vi "Test_PreloadNormalMsg_SendLowPriorityStop_StopAfterNormalMsg.vi"(8 "error in (no error)":errorcluster, 11 "TestCase in":refnum<class "TestPriorityStopMessage.lvclass">) -> (0 "error out":errorcluster, 3 "TestCase out":refnum<class "TestPriorityStopMessage.lvclass">)   [LabVIEW 2017, in "TestPriorityStopMessage.lvclass"]
uses:
  TestPriorityStopMessage.lvclass
  <vilib>/ActorFramework/Message Enqueuer/Message Priority.ctl
  <vilib>/ActorFramework/Message Enqueuer/Message Enqueuer.lvclass/Message Enqueuer.ctl
  Doubles/MessageCountsExecutions/MessageCountsExecutions.lvclass
  C:/Program Files (x86)/National Instruments/LabVIEW 2017/vi.lib/ActorFramework/Message/Message.lvclass
  Doubles/ActorBlockedUntilNotified/ActorBlockedUntilNotified.lvclass
  C:/Program Files (x86)/National Instruments/LabVIEW 2017/vi.lib/ActorFramework/Actor/Actor.lvclass
  <vilib>/ActorFramework/Stop Msg/Stop Msg.lvclass
  <vilib>/ActorFramework/Message Priority Queue/Priority Enqueue.vi
  <vilib>/ActorFramework/Actor/Actor.lvclass
  <vilib>/ActorFramework/Message Enqueuer/Message Enqueuer.lvclass
  Source/PriorityStopMessage/PriorityStopMessage.lvclass
panel:
  out "Msg Notification History":cluster{u32, "timed out?":bool}[](array[cluster])
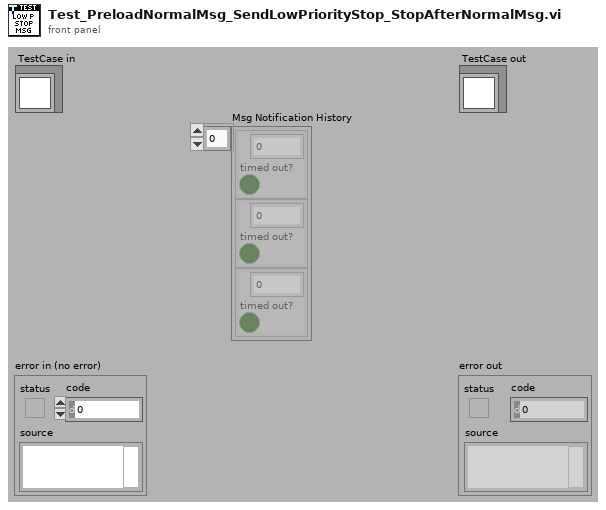
[diagram p1: front panel]
types:
  T1 = typedef "Actor Framework.lvlib/Message Enqueuer.lvclass/Message Priority.ctl" = enum16{"Low", "Normal", "High"}
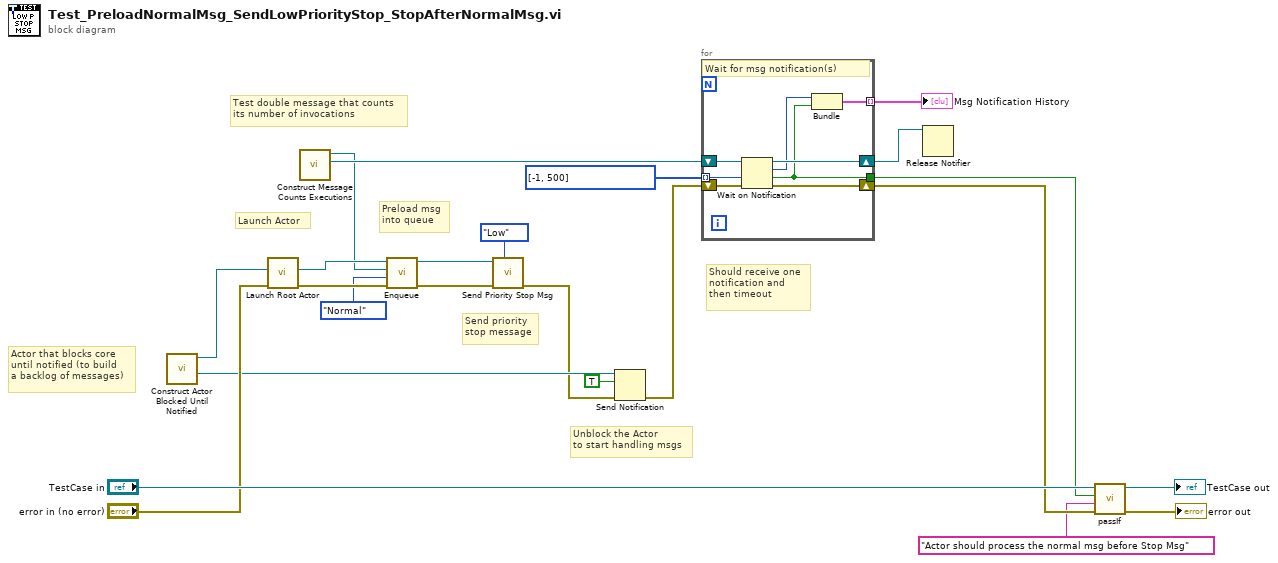
[diagram p0: block diagram]
diagram:
  # "Should receive one\nnotification and\nthen timeout"
  # "Send priority\nstop message"
  # "Preload msg\ninto queue"
  # "Unblock the Actor\nto start handling msgs"
  # "Actor that blocks core\nuntil notified (to build\na backlog of messages)"
  # "Test double message that counts\nits number of invocations"
  # "Launch Actor"
  n1 = call "Construct Actor Blocked Until Notified.vi"() -> ("Unblock Notifier"=w14:refnum<notifier>, "ActorBlockedUntilNotified"=w15:refnum<class "ActorBlockedUntilNotified.lvclass">)  [unwired: 10 in]
  n2 = call <vilib>:"Launch Root Actor.vi"("error in (no error)"="error in (no error)", "Actor"=w15) -> ("error out"=w18:errorcluster, "Actor's Enqueuer"=w11:refnum<class "Message Enqueuer.lvclass">)  [unwired: 8 in]
  n3 = call "Construct Message Counts Executions.vi"() -> ("Message Executions"=w19:refnum<notifier>, "CyclicMessageCountsCycles out"=w10:refnum<class "MessageCountsExecutions.lvclass">)  [unwired: 9 in, 1 out]
  n4 = call <vilib>:"Enqueue.vi"("error in (no error)"=w18, "Message Priority (Normal)"=Message_Priority."Normal" ("Message Priority"), "Message"=w10, "Message Enqueuer in"=w11) -> ("error out"=w12:errorcluster, "Message Enqueuer out"=w7:refnum<class "Message Enqueuer.lvclass">)  [unwired: 6 in]
  n5 = call "Send Priority Stop Msg.vi"("Message Priority (Normal)"=Message_Priority."Low", "error in (no error)"=w12, "Message Enqueuer"=w7) -> ("error out"=w8:errorcluster)  [unwired: 8 in]
  n6 = Send Notification(notification=TRUE, notifier=w14, error in (no error)=w8) -> (error out=w6:errorcluster)  [unwired: 1 out]
  n7 = for {
    shift-right: [w30] -> w5
    shift-left: w19 -> [w31]
    shift-right: [w28] -> w17
    shift-left: w6 -> [w29]
    tunnel: i32[] [-1, 500] -> [w27] mode=indexing
    tunnel: [w25] -> w1 mode=indexing
    tunnel: [w24] -> w2
    # "Wait for msg notification(s)"
    n8 = Wait on Notification(notifier=w31, timeout in ms (-1)=w27, error in (no error)=w29) -> (notifier out=w30:refnum<notifier>, notification=w26:u32, timed out?=w24:bool, error out=w28:errorcluster)  [unwired: 1 in]
    n9 = Bundle(w26, "timed out?"=w24) -> (w25:cluster{u32, "timed out?":bool})  [unwired: 1 in]
  }
  "Msg Notification History" <- w1
  n10 = Release Notifier(notifier=w5) -> ()  [unwired: 2 in, 3 out]
  n11 = call-dynamic "passIf.vi"("error in (no error)"=w17, "message (\"\")"="Actor should process the normal msg before Stop Msg" ("message (\"\")"), "pass"=w2, "TestCase in"="TestCase in") -> ("error out"=→"error out":errorcluster, "TestCase out"=→"TestCase out":refnum<class "TestPriorityStopMessage.lvclass">)  [unwired: 6 in]
